vi "Copy Set Default Value Multiple.vi"(11 "error in (no error)":errorcluster) -> (15 "error out":errorcluster)   [LabVIEW 2021, in "Converter.lvlib"]
uses:
  Converter.lvlib
  Path Functions/Path Functions.lvlib
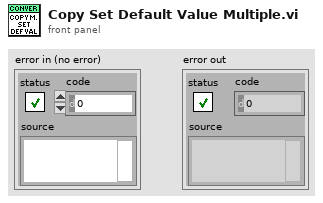
[diagram p1: front panel]
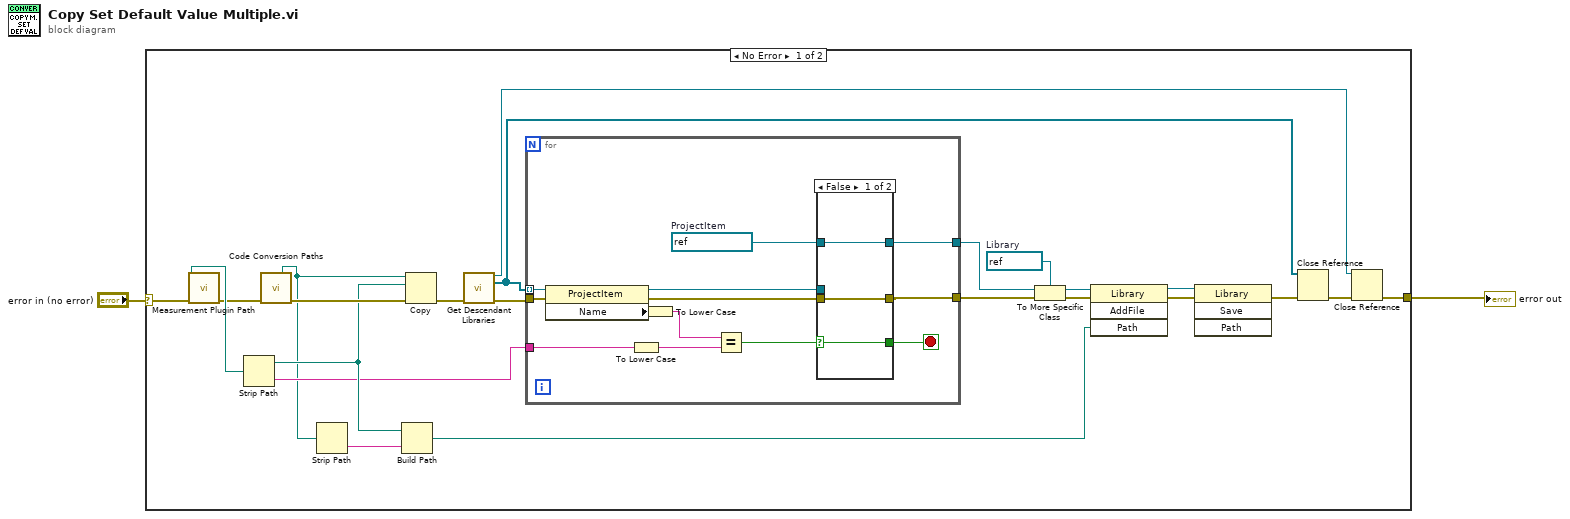
[diagram p0: block diagram]
diagram:
  n1 = case shown="No Error" "error in (no error)" {
    selector: "error in (no error)" -> [w12 w45]
    tunnel: [w16 w45] -> w2
    frame No Error {
      w4 = refnum<vi> refnum  # Library
      n2 = call "Measurement Plugin Path.vi"("error in (no error)"=w12) -> ("Measurement UI Lib"=w13:path, "error out"=w11:errorcluster)  [unwired: 2 in, 11 out]
      n3 = Strip Path(path=w13) -> (stripped path=w23:path, name=w22:string)
      n4 = call "Code Conversion Paths.vi"("error in (no error)"=w11) -> ("Deafult value setter VI"=w15:path, "error out"=w25:errorcluster)  [unwired: 6 in, 7 out]
      n5 = Strip Path(path=w15) -> (name=w14:string)  [unwired: 1 out]
      n6 = Build Path(base path=w23, name or relative path=w14) -> (appended path=w6:path)
      n7 = Copy(8:w25, 10:w23, 11:w15) -> (0:w10:errorcluster)  [unwired: 2 in, 2 out]
      n8 = call "Get Descendant Libraries.vi"("error in (no error)"=w10) -> ("Project out"=w17:refnum<vi>, "All Descendents"=w21:refnum<vi>[], "error out"=w24:errorcluster)  [unwired: 12 in]
      n9 = for {
        tunnel: w21 -> [w38] mode=indexing
        tunnel: [w31] -> w19
        tunnel: [w30] -> w7
        tunnel: w22 -> [w29]
        tunnel: w24 -> [w28]
        stop <- w32 stop-if-true
        w35 = refnum<vi> refnum  # ProjectItem
        n10 = property class="ProjectItem"(reference=w38, error in=w28) -> (reference out=w34:refnum<vi>, error out=w33:errorcluster, "Name"=w37:string)
        n11 = To Lower Case(string=w29) -> (all lower case string=w26:string)
        n12 = To Lower Case(string=w37) -> (all lower case string=w27:string)
        n13 = Equal?(x=w27, y=w26) -> (x = y?=w36:bool)
        n14 = case shown="False" w36 {
          selector: w36 -> [w40 w43]
          tunnel: w34 -> [_ w44]
          tunnel: [w39 w42] -> w30
          tunnel: [w41 w44] -> w31
          tunnel: w35 -> [w41 _]
          tunnel: [w40 w43] -> w32
          tunnel: w33 -> [w39 w42]
          frame False {
          }
          frame True {
          }
        }
      }
      n15 = To More Specific Class(target class=w4, reference=w19, error in=w7) -> (specific class reference=w3:refnum<vi>, error out=w5:errorcluster)
      n16 = invoke class="Library" method="AddFile"(reference=w3, error in=w5, "Path"=w6) -> (reference out=w9:refnum<vi>, error out=w8:errorcluster)  [unwired: 1 in, 2 out]
      n17 = invoke class="Library" method="Save"(reference=w9, error in=w8) -> (error out=w18:errorcluster)  [unwired: 2 in, 3 out]
      n18 = Close Reference(reference=w21, error in (no error)=w18) -> (error out=w20:errorcluster)
      n19 = Close Reference(reference=w17, error in (no error)=w20) -> (error out=w16:errorcluster)
    }
    frame Error {
    }
  }
  "error out" <- w2
